vi "CRYGraph Cluster Init.vi"(10 "Data View Number":i32, 11 "Queue Name":string) -> ()   [LabVIEW 2013]
uses:
  Control/CRYGraph Event.ctl
  CRYData View Global.vi
panel:
  # "Initialize Graph Cluster"
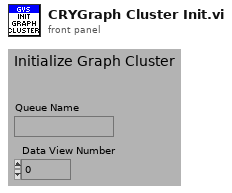
[diagram p1: front panel]
types:
  T1 = typedef "CRYGraph Event.ctl" = cluster{"EvenName":string, "TitleName":string, "GraphName":string, "GraphType":string, "Data":variant, "Queue Name":string, "DataView Number":i32}
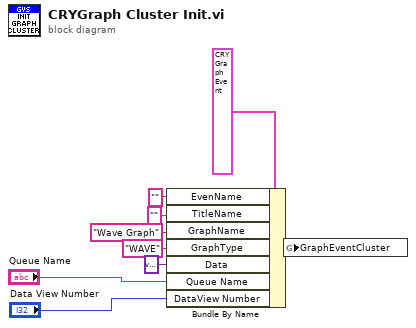
[diagram p0: block diagram]
diagram:
  n1 = Bundle By Name(cluster=T1 {"EvenName"="", "TitleName"="", "GraphName"="", "GraphType"="", "Data"=variant, "Queue Name"="", "DataView Number"=0} ("GraphEventCluster"), "EvenName"="", "TitleName"="", "GraphName"="Wave Graph" ("GraphType"), "GraphType"="WAVE" ("DataType"), "Data"=variant, "Queue Name"="Queue Name", "DataView Number"="Data View Number") -> (w9:T1)
  n2 = global write "CRYData View Global.vi" "GraphEventCluster"(w9) -> ()
